vi "oa_Create Indice Tacho Pulse Counter.vi"(9 "length":i32, 10 "reset?":bool) -> (1 "tacho pulse passed last round":i32, 2 "tacho pulse passed":i32)   [LabVIEW 2017]
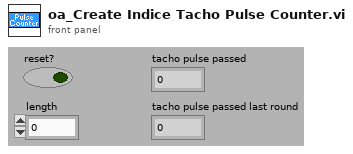
[diagram p1: front panel]
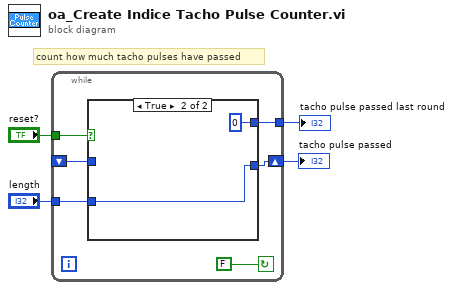
[diagram p0: block diagram]
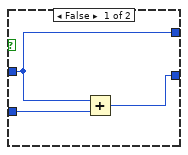
[diagram p2: hidden frame]
diagram:
  # "count how much tacho pulses have passed"
  n1 = while {
    tunnel: "reset?" -> [w9]
    tunnel: "length" -> [w8]
    shift-right: [w7] -> w2
    shift-left: _ -> [w6]
    tunnel: [w5] -> w1
    stop <- FALSE continue-if-true
    n2 = case shown="True" w9 {
      tunnel: w8 -> [w13 w14]
      tunnel: [w12 w14] -> w7
      tunnel: w6 -> [w11 _]
      tunnel: [w11 0] -> w5
      frame False {
        n3 = Add(x=w11, y=w13) -> (x+y=w12:i32)
      }
      frame True {
      }
    }
  }
  "tacho pulse passed" <- w2
  "tacho pulse passed last round" <- w1
